vi "LEP_RV_Test.vi"(8 "error in (no error)":errorcluster) -> (0 "error out":errorcluster)   [LabVIEW 2011]
doc: "Runs the embedded application on a console located in the <B>Build Path</B> directory ."
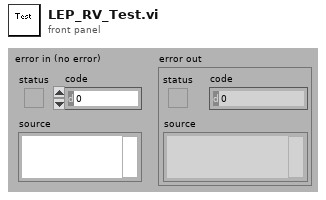
[diagram p1: front panel]
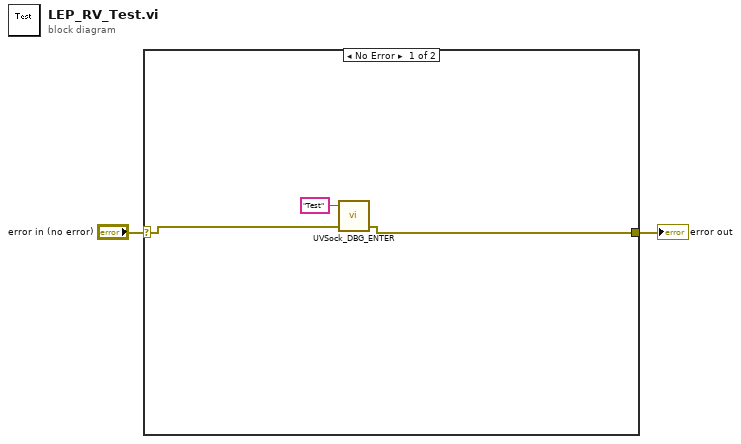
[diagram p0: block diagram]
diagram:
  n1 = case shown="No Error" "error in (no error)" {
    selector: "error in (no error)" -> [w5 w6]
    tunnel: [w4 w6] -> w1
    frame No Error {
      n2 = call "UVSock_DBG_ENTER.vi"("error in (no error)"=w5, "Target"="Test") -> ("error out"=w4:errorcluster)  [unwired: 3 in]
    }
    frame Error {
    }
  }
  "error out" <- w1
